vi "Delete Message.vi"   [LabVIEW 2015, in "NI_AWS_SQS.lvclass"]
uses:
  NI_AWS_SQS.lvclass
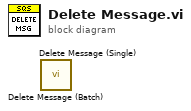
[diagram p0: block diagram]
diagram:
  n1 = call "Delete Message (Batch).vi"() -> ()  [unwired: 10 in, 2 out]
  n2 = call "Delete Message (Single).vi"() -> ()  [unwired: 10 in, 2 out]
